vi "停止判断1.vi"(6 "重置？":bool, 7 "反转？":bool, 8 "error in (no error)":errorcluster caption="错误输入（无错误）", 9 "反转判断条件1":T1, 10 "传感器数据":dbl[](array[numeric]), 11 "Message Queues":T2 caption="消息队列") -> (0 "error out":errorcluster caption="错误输出")   [LabVIEW 2015, in "Action.lvlib"]
uses:
  Action.lvlib
  support/Message Queue/All Message Queues.ctl
  support/Message Queue/Message Cluster.ctl
  support/Message Queue/Enqueue Message (Single).vi
  support/Message Queue/Message Queue.lvlib
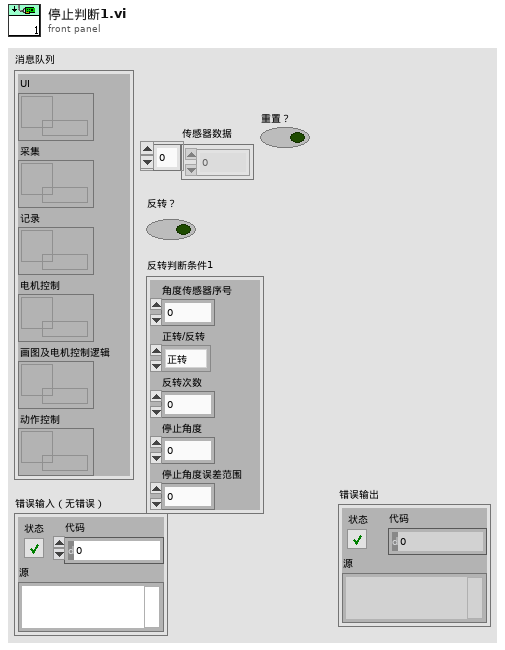
[diagram p1: front panel]
types:
  T1 = typedef "Action.lvlib/停止判断条件1.ctl" = cluster{"角度传感器序号":i32, "正转/反转":enum16{"正转", "反转"}, "反转次数":i32, "停止角度":dbl, "停止角度误差范围":dbl}
  T2 = typedef "Message Queue.lvlib/All Message Queues.ctl" = cluster{"UI":refnum<queue>, "Acquisition":refnum<queue>, "Logging":refnum<queue>, "MotorCtrl":refnum<queue>, "plot logic":refnum<queue>, "Action Control":refnum<queue>}
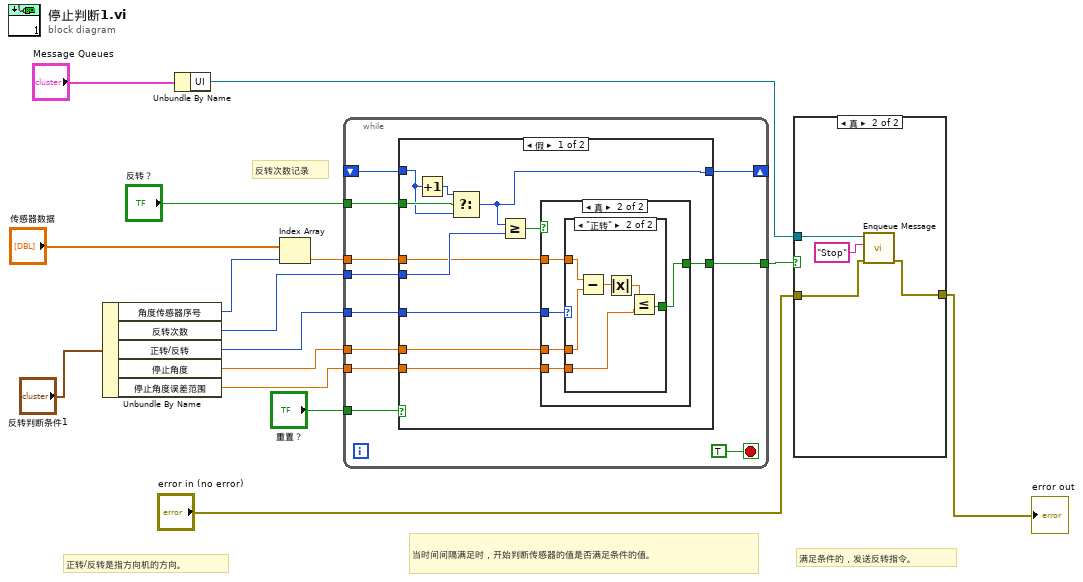
[diagram p0: block diagram]
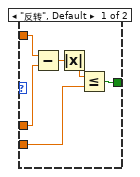
[diagram p4: hidden frame]
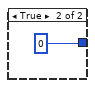
[diagram p5: hidden frame]
diagram:
  # "正转/反转是指方向机的方向。"
  # "满足条件的，发送反转指令。"
  # "当时间间隔满足时，开始判断传感器的值是否满足条件的值。"
  # "反转次数记录"
  n1 = Unbundle By Name("反转判断条件1") -> ("角度传感器序号"=w3:i32, "反转次数"=w12:i32, "正转/反转"=w2:enum16{"正转", "反转"}, "停止角度"=w10:dbl, "停止角度误差范围"=w9:dbl)
  n2 = Unbundle By Name("Message Queues") -> ("UI"=w7:refnum<queue>)
  n3 = Index Array(array="传感器数据", index=w3) -> (element=w11:dbl)
  n4 = while {
    tunnel: w12 -> [w26]
    tunnel: w11 -> [w25]
    tunnel: w10 -> [w24]
    shift-right: [w23] -> _
    shift-left: _ -> [w17]
    tunnel: w9 -> [w22]
    tunnel: [w21] -> w8
    tunnel: "反转？" -> [w19]
    tunnel: w2 -> [w18]
    tunnel: "重置？" -> [w16]
    stop <- TRUE stop-if-true
    n5 = case shown="假" w16 {
      tunnel: w26 -> [w33 _]
      tunnel: w25 -> [w31 _]
      tunnel: w24 -> [w29 _]
      tunnel: [w34 0] -> w23
      tunnel: w17 -> [w35 _]
      tunnel: w22 -> [w28 _]
      tunnel: [w27 _] -> w21
      tunnel: w19 -> [w37 _]
      tunnel: w18 -> [w30 _]
      frame False {
        n6 = Increment(x=w35) -> (x+1=w36:i32)
        n7 = Select(t=w36, s=w37, f=w35) -> (s? t:f=w34:i32)
        n8 = Greater Or Equal?(x=w34, y=w33) -> (x >= y?=w32:bool)
        n9 = case shown="真" w32 {
          tunnel: w31 -> [_ w42]
          tunnel: w30 -> [_ w38]
          tunnel: w29 -> [_ w41]
          tunnel: w28 -> [_ w40]
          tunnel: [_ w39] -> w27
          frame False {
          }
          frame True {
            n10 = case shown="\"正转\"" w38 {
              tunnel: w42 -> [w48 w54]
              tunnel: w41 -> [w47 w53]
              tunnel: w40 -> [w46 w51]
              tunnel: [w45 w49] -> w39
              frame "反转", Default {
                n11 = Subtract(x=w48, y=w47) -> (x-y=w44:dbl)
                n12 = Absolute Value(x=w44) -> (abs(x)=w43:dbl)
                n13 = Less Or Equal?(x=w43, y=w46) -> (x <= y?=w45:bool)
              }
              frame "正转" {
                n14 = Subtract(x=w54, y=w53) -> (x-y=w52:dbl)
                n15 = Absolute Value(x=w52) -> (abs(x)=w50:dbl)
                n16 = Less Or Equal?(x=w50, y=w51) -> (x <= y?=w49:bool)
              }
            }
          }
        }
      }
      frame True {
      }
    }
  }
  n17 = case shown="真" w8 {
    tunnel: w7 -> [_ w60]
    tunnel: "error in (no error)" -> [w56 w59]
    tunnel: [w56 w58] -> w5
    frame False {
    }
    frame True {
      n18 = call-poly "Enqueue Message.vi"("error in (no error)"=w59, "Message"="Stop", "Message Queue"=w60) -> ("error out"=w58:errorcluster)  [unwired: 7 in, 1 out]
    }
  }
  "error out" <- w5
